vi "CalcState.vi"(0 "reference in":refnum<class "NeedleValve.lvclass">, 11 "error in (no error)":errorcluster) -> (4 "reference out":refnum<class "NeedleValve.lvclass">, 15 "error out":errorcluster)   [LabVIEW 2019, in "NeedleValve.lvclass"]
uses:
  NeedleValve.lvclass
  NeedleValve.lvclass/NeedleValve.ctl
  TypeDef/Needle Valve State.ctl
  modbus engine custom/MB_ENGINE_class/cmd enum.ctl
  Cmd.ctl
  8527a047-540e-4be4-8d90-8e4a228dfd96.vi
  7786ce6c-c59e-4fbc-9e94-2933324a4a28.vi
  modbus engine custom/MB_ENGINE_class/MB_ENGINE.lvclass
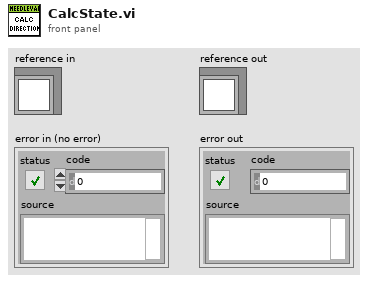
[diagram p1: front panel]
types:
  T1 = typedef "Needle Valve State.ctl" = enum16{"STOPED", "CLOSED", "OPENED", "OPENING", "CLOSING", "FULL_CLOSE", "PREP_OPEN"}
  T2 = typedef "NeedleValve.lvclass/Cmd.ctl" = enum16{"Open", "Close", "Stop", "Prep open"}
  T3 = typedef "Needle Valve Data.ctl" = cluster{"Engine State":T4, "StateValveModbus":T1, "Alarms":T5, "RAW":i32, "Angele":dbl, "Step":i32, "Encoder":i32, "Kinematic":T6, "Limits":T7, "EncoderMax":i32, "Counter Max Dont Update":i32, "EncoderMin":i32, "Counter Min Dont Update":i32, "Prepere Counter":i32, "STEP INIT":i32, "offset - Angel":dbl}
  T4 = typedef "MB_ENGINE.lvclass/Engine State.ctl" = u16
  T5 = typedef "MB_ENGINE.lvclass/Engine Alarms.ctl" = cluster{"OL":bool, "TF":bool, "STL":bool, "OCP":bool, "CPUV":bool, "UVLO":bool, "SPI_ERROR":bool, "Fault":bool, "OL 2":bool, "TF 2":bool, "STL 2":bool, "OCP 2":bool, "CPUV 2":bool, "UVLO 2":bool, "reserved":bool, "InitDone":bool}
  T6 = typedef "MB_ENGINE.lvclass/Settings.ctl" = cluster{"ACC Steps Per Sec^2":u16, "DEC Steps Per Sec^2":u16, "Min Velosity Step Per Sec":u16, "Max Velosity Step Per Sec":u16, "MicroStep":u16}
  T7 = typedef "MB_ENGINE.lvclass/Limits Status.ctl" = cluster{"Fault 2 Switch":bool, "Fault 1 Switch":bool, "Center(Home)":bool, "Lower Limit":bool, "Upper Limit":bool}
  T8 = typedef "MB_ENGINE.lvclass/cmd enum.ctl" = u16
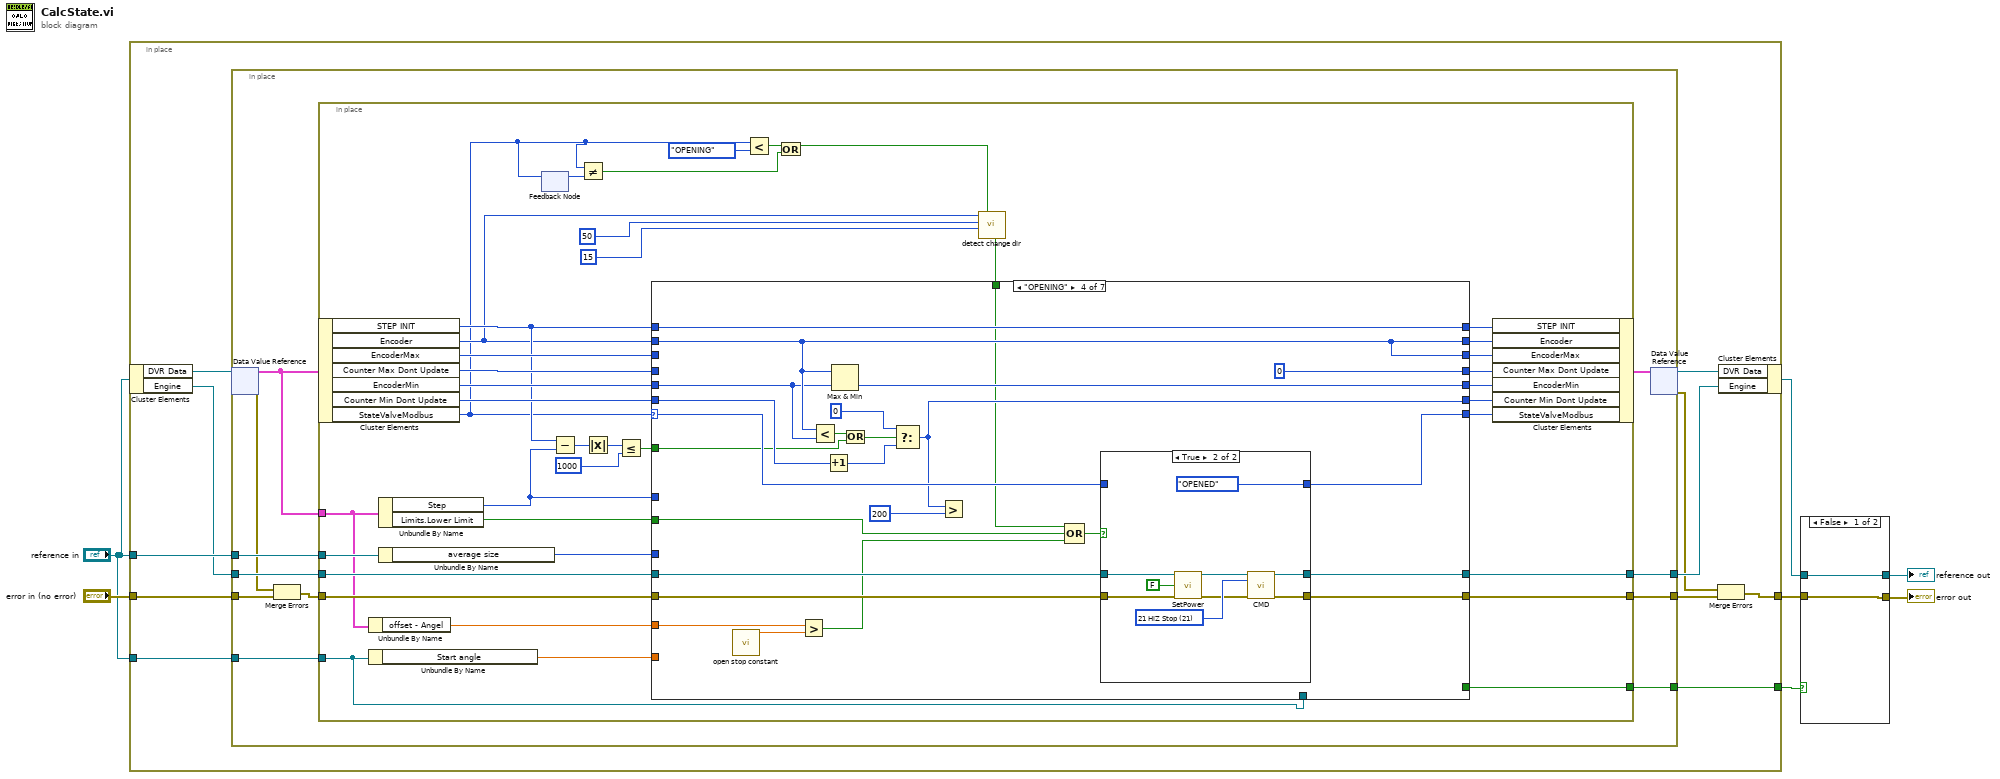
[diagram p0: block diagram]
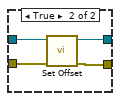
[diagram p2: hidden frame]
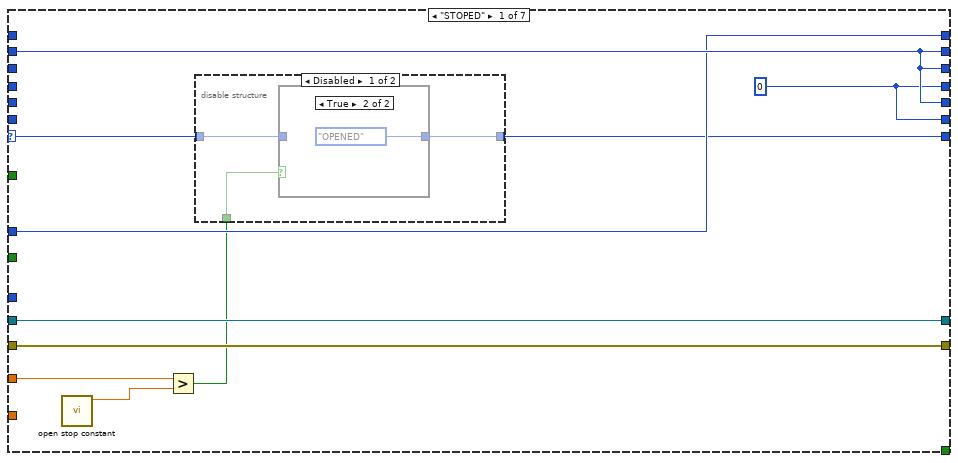
[diagram p3: hidden frame]
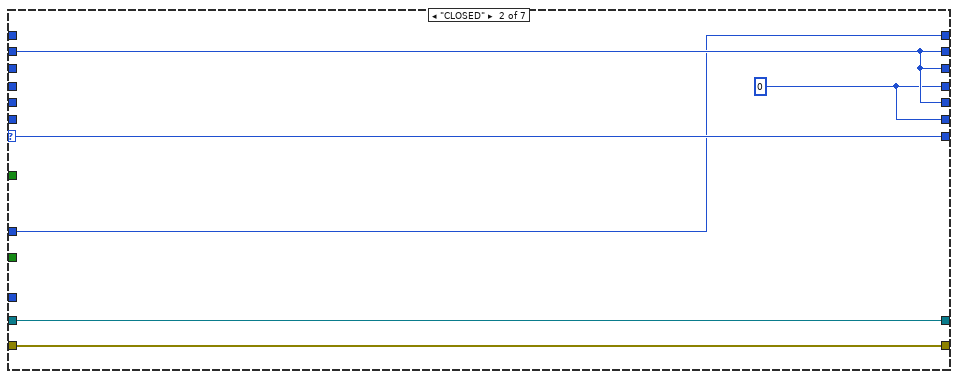
[diagram p6: hidden frame]
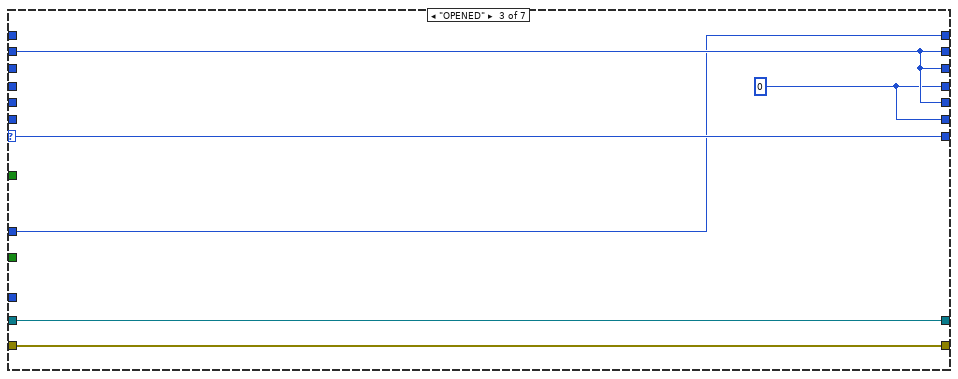
[diagram p7: hidden frame]
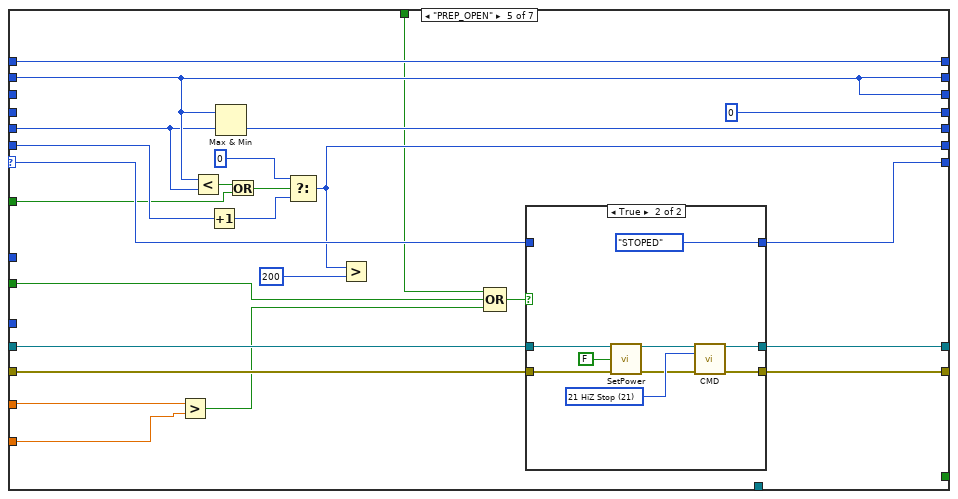
[diagram p9: hidden frame]
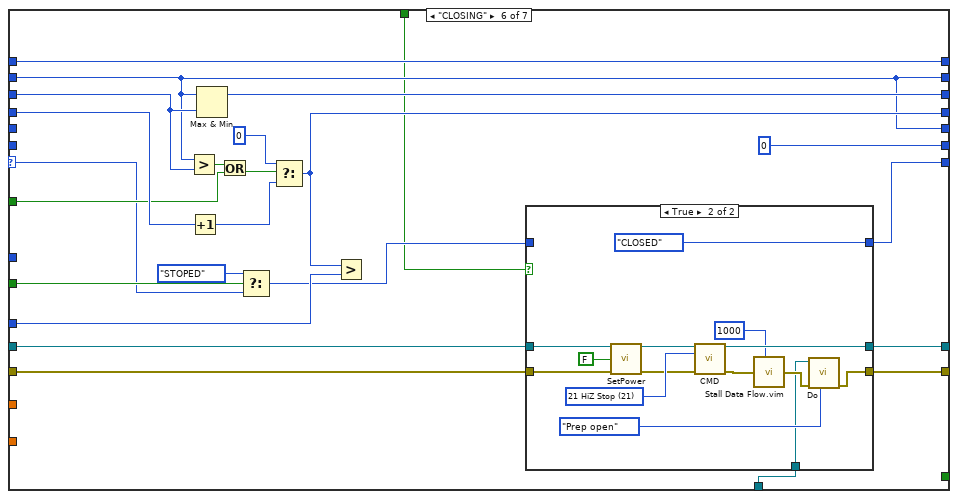
[diagram p11: hidden frame]
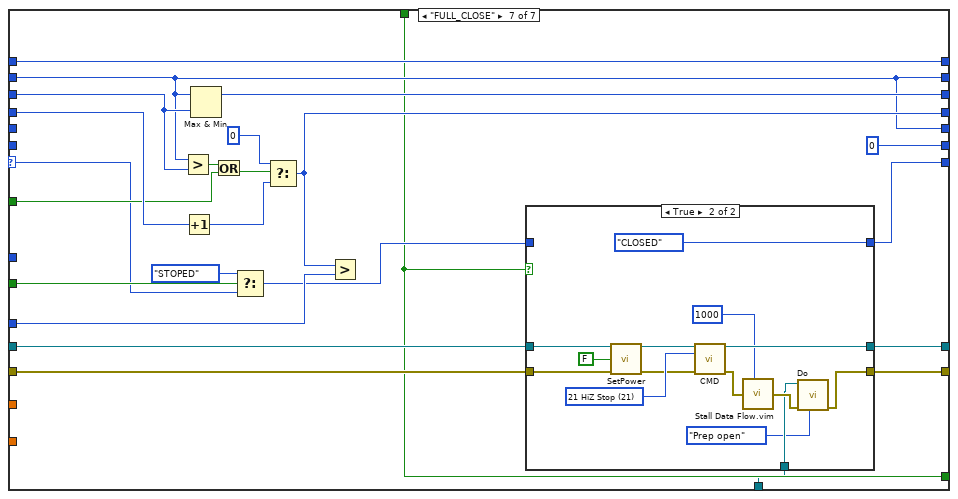
[diagram p13: hidden frame]
diagram:
  n1 = in-place {
    in-place-border: "error in (no error)" -> [w18]
    in-place-border: [w11] -> w6
    in-place-border: "reference in" -> [w15]
    in-place-border: [w9] -> w2
    in-place-border: "reference in" -> [w8]
    n2 = in-place-cluster #1("reference in") -> ("DVR Data"=w16:refnum<data-value>, "Engine"=w14:refnum<class "MB_ENGINE.lvclass">)
    n3 = in-place {
      in-place-border: w18 -> [w29]
      in-place-border: [w28] -> w17
      in-place-border: w15 -> [w26]
      in-place-border: w14 -> [w25]
      in-place-border: [w24] -> w13
      in-place-border: [w20] -> w9
      in-place-border: w8 -> [w19]
      n4 = in-place-dvr #2(w16) -> (w27:T3, w21:errorcluster)
      n5 = Merge Errors(w21, w29) -> (w22:errorcluster)
      n6 = in-place {
        in-place-border: w27 -> [w45]
        in-place-border: w22 -> [w62]
        in-place-border: [w61] -> w28
        in-place-border: w26 -> [w49]
        in-place-border: w25 -> [w47]
        in-place-border: [w46] -> w24
        in-place-border: [w43] -> w20
        in-place-border: w19 -> [w34]
        n7 = in-place-cluster #3(w27) -> ("STEP INIT"=w42:i32, "Encoder"=w39:i32, "EncoderMax"=w65:i32, "Counter Max Dont Update"=w64:i32, "EncoderMin"=w60:i32, "Counter Min Dont Update"=w59:i32, "StateValveModbus"=w32:T1)
        n8 = Unbundle By Name(w45) -> ("offset - Angel"=w44:dbl)
        n9 = Unbundle By Name(w34) -> ("Start angle"=w35:dbl)
        n10 = Unbundle By Name(w45) -> ("Step"=w50:i32, "Limits.Lower Limit"=w56:bool)
        n11 = Unbundle By Name(w49) -> ("average size"=w48:i32)
        n12 = feedback-in #4(w32) -> ()
        n13 = feedback #4() -> (w33:T1)  [unwired: 1 in]
        n14 = Subtract(x=w42, y=w50) -> (x-y=w53:i32)
        n15 = Not Equal?(x=w32, y=w33) -> (x != y?=w30:bool)
        n16 = Absolute Value(x=w53) -> (abs(x)=w54:i32)
        n17 = Less Or Equal?(x=w54, y=1000) -> (x <= y?=w51:bool)
        n18 = Less?(x=w32, y=Needle_Valve_State."OPENING") -> (x < y?=w36:bool)
        n19 = Or(x=w36, y=w30) -> (x .or. y?=w31:bool)
        n20 = call "detect change dir.vi"("reset"=w31, "cont stop"=u32 15, "max dont change"=50, "in"=w39) -> ("stop"=w38:bool)  [unwired: 3 in, 4 out]
        n21 = case shown="\"OPENING\"" w32 {
          selector: w32 -> [w70 w90 w96 w118 w155 w175 w216]
          tunnel: [w76 w87 w93 w111 w148 w181 w222] -> w68
          tunnel: w39 -> [w76 w87 w93 w111 w148 w181 w222]
          tunnel: [w69 w90 w96 w117 w154 w186 w227] -> w63
          tunnel: [w76 w87 w93 w111 w148 w194 w235] -> w67
          tunnel: [w75 w86 w92 0 ("Counter Max Dont Update") 0 ("Counter Max Dont Update") w188 w229] -> w66
          tunnel: w65 -> [_ _ _ _ _ w191 w232]
          tunnel: w64 -> [_ _ _ _ _ w190 w231]
          tunnel: w48 -> [_ _ _ _ _ w187 w228]
          tunnel: w47 -> [w78 w89 w95 w116 w153 w185 w226]
          tunnel: [w78 w89 w95 w115 w152 w184 w225] -> w46
          tunnel: w62 -> [w77 w88 w94 w114 w151 w183 w224]
          tunnel: [w77 w88 w94 w113 w150 w182 w223] -> w61
          tunnel: w60 -> [_ _ _ w108 w145 _ _]
          tunnel: w59 -> [_ _ _ w110 w147 _ _]
          tunnel: [w76 w87 w93 w109 w146 w181 w222] -> w58
          tunnel: [w75 w86 w92 w107 w144 0 ("Counter Max Dont Update") 0 ("Counter Max Dont Update")] -> w57
          tunnel: w56 -> [_ _ _ w104 w141 w176 w217]
          tunnel: w50 -> [w74 w85 w91 _ _ _ _]
          tunnel: [w74 w85 w91 w102 w139 w179 w220] -> w55
          tunnel: w42 -> [_ _ _ w102 w139 w179 w220]
          tunnel: w51 -> [_ _ _ w101 w138 w177 w218]
          tunnel: w44 -> [w72 _ _ w100 w135 _ _]
          tunnel: [_ _ _ _ _ _ w213] -> w43
          tunnel: w38 -> [_ _ _ w97 w136 w172 w213]
          tunnel: w35 -> [_ _ _ _ w134 _ _]
          tunnel: w34 -> [_ _ _ _ _ w171 w212]
          frame "STOPED" {
            w75 = 0 ("Counter Max Dont Update")
            n22 = call "open stop constant.vi"() -> ("angle"=w73:dbl)  [unwired: 11 in]
            n23 = Greater?(x=w72, y=w73) -> (0:w71:bool)
            n24 = disable-structure shown="Disabled" {
              disable-tunnel: w71 -> [w81 _]
              disable-tunnel: w70 -> [w80 w84]
              disable-tunnel: [w79 w84] -> w69
              frame Disabled {
                n25 = case shown="True" w81 {
                  tunnel: w80 -> [w82 _]
                  tunnel: [w82 Needle_Valve_State."OPENED" ("StateValveModbus")] -> w79
                  frame False {
                  }
                  frame True {
                  }
                }
              }
              frame Enabled {
              }
            }
          }
          frame "CLOSED" {
            w86 = 0 ("Counter Max Dont Update")
          }
          frame "OPENED" {
            w92 = 0 ("Counter Max Dont Update")
          }
          frame "OPENING" {
            n26 = call "open stop constant.vi"() -> ("angle"=w98:dbl)  [unwired: 11 in]
            n27 = Greater?(x=w100, y=w98) -> (0:w99:bool)
            n28 = Less?(x=w111, y=w108) -> (x < y?=w120:bool)
            n29 = Increment(x=w110) -> (x+1=w119:i32)
            n30 = Max & Min(x=w111, y=w108) -> (min(x,y)=w109:i32)  [unwired: 1 out]
            n31 = Or(x=w120, y=w101) -> (x .or. y?=w103:bool)
            n32 = Select(t=0, s=w103, f=w119) -> (s? t:f=w107:i32)
            n33 = Greater?(x=w107, y=200) -> ()  [unwired: 1 out]
            n34 = Compound Arithmetic op=OR(w97, w104, w99) -> (w105:bool)
            n35 = case shown="True" w105 {
              tunnel: w118 -> [w124 _]
              tunnel: [w124 Needle_Valve_State."OPENED" ("StateValveModbus")] -> w117
              tunnel: w116 -> [w123 w128]
              tunnel: [w123 w127] -> w115
              tunnel: w114 -> [w122 w126]
              tunnel: [w122 w125] -> w113
              frame False {
              }
              frame True {
                w132 = T8 21 items=["0 Idle"=0, "1 GoTo Absolute Position"=1, "2 GoTo Relative"=2, "10 GoTo Home Position"=10, "11 Set Home Position"=11, "12 Set FindHome Mode"=12, "13 Reset FindHome Mode"=13, "14 Get FindHome State"=14, "20 Hard Stop"=20, "21 HiZ Stop"=21, "22 Soft Stop"=22, "30 Clear Fault"=30, "40 Encoder Set Home"=40, "70 Driver Init"=70] ("cmd to write")
                n36 = call "SetPower.vi"("class data in"=w128, "On"=FALSE, "error in (no error)"=w126) -> ("class data out"=w129:refnum<class "MB_ENGINE.lvclass">, "error out"=w130:errorcluster)  [unwired: 11 in]
                n37 = call "CMD.vi"("class data in"=w129, "cmd to write"=w132, "error in (no error)"=w130) -> ("class data out"=w127:refnum<class "MB_ENGINE.lvclass">, "error out"=w125:errorcluster)  [unwired: 11 in]
              }
            }
          }
          frame "PREP_OPEN" {
            n38 = Greater?(x=w135, y=w134) -> (0:w137:bool)
            n39 = Less?(x=w148, y=w145) -> (x < y?=w157:bool)
            n40 = Increment(x=w147) -> (x+1=w156:i32)
            n41 = Max & Min(x=w148, y=w145) -> (min(x,y)=w146:i32)  [unwired: 1 out]
            n42 = Or(x=w157, y=w138) -> (x .or. y?=w140:bool)
            n43 = Select(t=0, s=w140, f=w156) -> (s? t:f=w144:i32)
            n44 = Greater?(x=w144, y=200) -> ()  [unwired: 1 out]
            n45 = Compound Arithmetic op=OR(w136, w141, w137) -> (w142:bool)
            n46 = case shown="True" w142 {
              tunnel: w155 -> [w161 _]
              tunnel: [w161 Needle_Valve_State."STOPED" ("StateValveModbus")] -> w154
              tunnel: w153 -> [w160 w165]
              tunnel: [w160 w164] -> w152
              tunnel: w151 -> [w159 w163]
              tunnel: [w159 w162] -> w150
              frame False {
              }
              frame True {
                w169 = T8 21 items=["0 Idle"=0, "1 GoTo Absolute Position"=1, "2 GoTo Relative"=2, "10 GoTo Home Position"=10, "11 Set Home Position"=11, "12 Set FindHome Mode"=12, "13 Reset FindHome Mode"=13, "14 Get FindHome State"=14, "20 Hard Stop"=20, "21 HiZ Stop"=21, "22 Soft Stop"=22, "30 Clear Fault"=30, "40 Encoder Set Home"=40, "70 Driver Init"=70] ("cmd to write")
                n47 = call "SetPower.vi"("class data in"=w165, "On"=FALSE, "error in (no error)"=w163) -> ("class data out"=w166:refnum<class "MB_ENGINE.lvclass">, "error out"=w167:errorcluster)  [unwired: 11 in]
                n48 = call "CMD.vi"("class data in"=w166, "cmd to write"=w169, "error in (no error)"=w167) -> ("class data out"=w164:refnum<class "MB_ENGINE.lvclass">, "error out"=w162:errorcluster)  [unwired: 11 in]
              }
            }
          }
          frame "CLOSING" {
            n49 = Greater?(x=w181, y=w191) -> (0:w192:bool)
            n50 = Increment(x=w190) -> (x+1=w189:i32)
            n51 = Max & Min(x=w181, y=w191) -> (max(x,y)=w194:i32)  [unwired: 1 out]
            n52 = Or(x=w192, y=w177) -> (x .or. y?=w178:bool)
            n53 = Select(t=Needle_Valve_State."STOPED", s=w176, f=w175) -> (s? t:f=w174:T1)
            n54 = Select(t=0, s=w178, f=w189) -> (s? t:f=w188:i32)
            n55 = Greater?(x=w188, y=w187) -> ()  [unwired: 1 out]
            n56 = case shown="True" w172 {
              tunnel: w174 -> [w197 _]
              tunnel: [w197 Needle_Valve_State."CLOSED" ("StateValveModbus")] -> w186
              tunnel: w185 -> [w196 w206]
              tunnel: [w196 w205] -> w184
              tunnel: w183 -> [w195 w204]
              tunnel: [w195 w200] -> w182
              tunnel: w171 -> [_ w199]
              frame False {
              }
              frame True {
                w210 = T8 21 items=["0 Idle"=0, "1 GoTo Absolute Position"=1, "2 GoTo Relative"=2, "10 GoTo Home Position"=10, "11 Set Home Position"=11, "12 Set FindHome Mode"=12, "13 Reset FindHome Mode"=13, "14 Get FindHome State"=14, "20 Hard Stop"=20, "21 HiZ Stop"=21, "22 Soft Stop"=22, "30 Clear Fault"=30, "40 Encoder Set Home"=40, "70 Driver Init"=70] ("cmd to write")
                n57 = call "SetPower.vi"("class data in"=w206, "On"=FALSE, "error in (no error)"=w204) -> ("class data out"=w207:refnum<class "MB_ENGINE.lvclass">, "error out"=w208:errorcluster)  [unwired: 11 in]
                n58 = call "CMD.vi"("class data in"=w207, "cmd to write"=w210, "error in (no error)"=w208) -> ("class data out"=w205:refnum<class "MB_ENGINE.lvclass">, "error out"=w203:errorcluster)  [unwired: 11 in]
                n59 = call "Stall Data Flow.vim"("value in"=w203, "milliseconds to wait"=u32 1000) -> ("value out"=w202:errorcluster)  [unwired: 1 out]
                n60 = call "Do.vi"("Cmd"=Cmd."Prep open", "error in (no error)"=w202, "NeedleValve in"=w199) -> ("error out"=w200:errorcluster)  [unwired: 7 in, 1 out]
              }
            }
          }
          frame "FULL_CLOSE" {
            n61 = Greater?(x=w222, y=w232) -> (0:w233:bool)
            n62 = Increment(x=w231) -> (x+1=w230:i32)
            n63 = Max & Min(x=w222, y=w232) -> (max(x,y)=w235:i32)  [unwired: 1 out]
            n64 = Or(x=w233, y=w218) -> (x .or. y?=w219:bool)
            n65 = Select(t=Needle_Valve_State."STOPED", s=w217, f=w216) -> (s? t:f=w215:T1)
            n66 = Select(t=0, s=w219, f=w230) -> (s? t:f=w229:i32)
            n67 = Greater?(x=w229, y=w228) -> ()  [unwired: 1 out]
            n68 = case shown="True" w213 {
              tunnel: w215 -> [w238 _]
              tunnel: [w238 Needle_Valve_State."CLOSED" ("StateValveModbus")] -> w227
              tunnel: w226 -> [w237 w247]
              tunnel: [w237 w246] -> w225
              tunnel: w224 -> [w236 w245]
              tunnel: [w236 w242] -> w223
              tunnel: w212 -> [_ w241]
              frame False {
              }
              frame True {
                w251 = T8 21 items=["0 Idle"=0, "1 GoTo Absolute Position"=1, "2 GoTo Relative"=2, "10 GoTo Home Position"=10, "11 Set Home Position"=11, "12 Set FindHome Mode"=12, "13 Reset FindHome Mode"=13, "14 Get FindHome State"=14, "20 Hard Stop"=20, "21 HiZ Stop"=21, "22 Soft Stop"=22, "30 Clear Fault"=30, "40 Encoder Set Home"=40, "70 Driver Init"=70] ("cmd to write")
                n69 = call "SetPower.vi"("class data in"=w247, "On"=FALSE, "error in (no error)"=w245) -> ("class data out"=w248:refnum<class "MB_ENGINE.lvclass">, "error out"=w249:errorcluster)  [unwired: 11 in]
                n70 = call "CMD.vi"("class data in"=w248, "cmd to write"=w251, "error in (no error)"=w249) -> ("class data out"=w246:refnum<class "MB_ENGINE.lvclass">, "error out"=w243:errorcluster)  [unwired: 11 in]
                n71 = call "Stall Data Flow.vim"("value in"=w243, "milliseconds to wait"=u32 1000) -> ("value out"=w244:errorcluster)  [unwired: 1 out]
                n72 = call "Do.vi"("Cmd"=Cmd."Prep open", "error in (no error)"=w244, "NeedleValve in"=w241) -> ("error out"=w242:errorcluster)  [unwired: 7 in, 1 out]
              }
            }
          }
        }
        n73 = in-place-cluster #3("STEP INIT"=w55, "Encoder"=w68, "EncoderMax"=w67, "Counter Max Dont Update"=w66, "EncoderMin"=w58, "Counter Min Dont Update"=w57, "StateValveModbus"=w63) -> (w23:T3)
      }
      n74 = in-place-dvr #2(w23) -> (w12:refnum<data-value>, w10:errorcluster)
    }
    n75 = Merge Errors(w10, w17) -> (w11:errorcluster)
    n76 = in-place-cluster #1("DVR Data"=w12, "Engine"=w13) -> (w4:refnum<class "NeedleValve.lvclass">)
  }
  n77 = case shown="False" w2 {
    tunnel: w6 -> [w253 w258]
    tunnel: [w253 w257] -> w5
    tunnel: w4 -> [w254 w256]
    tunnel: [w254 w255] -> w3
    frame False {
    }
    frame True {
      n78 = call "Set Offset.vi"("error in (no error)"=w258, "NeedleValve in"=w256) -> ("error out"=w257:errorcluster, "NeedleValve out"=w255:refnum<class "NeedleValve.lvclass">)  [unwired: 8 in]
    }
  }
  "reference out" <- w3
  "error out" <- w5
